vi "mp285_SetVelRes_velres2str.vi"(1 "速度":dbl, 2 "精度":u16(ring)=10 items=["Low (10microsteps/step)", "High (50microsteps/step)"]) -> (0 "发送至串口的字符串":string)   [LabVIEW 2018]
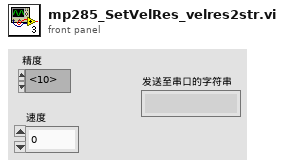
[diagram p1: front panel]
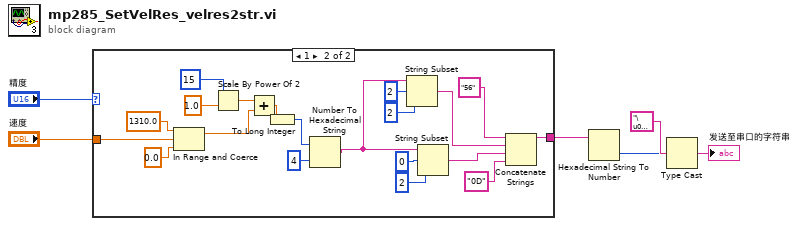
[diagram p0: block diagram]
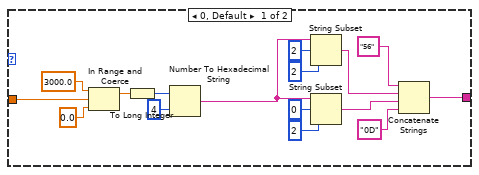
[diagram p2: hidden frame]
diagram:
  n1 = case shown="1" "精度" {
    tunnel: "速度" -> [w20 w42]
    tunnel: [w15 w30] -> w3
    frame 0, Default {
      n2 = In Range and Coerce(upper limit=3000.0 ("上限"), x=w20, lower limit=0.0 ("下限")) -> (coerced(x)=w19:dbl)  [unwired: 1 out]
      n3 = To Long Integer(number=w19) -> (32bit integer=w7:i32)
      n4 = Number To Hexadecimal String(1:i16 4 ("宽度(-)"), 2:w7) -> (0:w8:string)
      n5 = String Subset(string=w8, offset (0)=2 ("偏移量(0)"), length (rest)=2 ("长度（剩余）")) -> (substring=w10:string)
      n6 = String Subset(string=w8, offset (0)=0 ("偏移量(0)"), length (rest)=2 ("长度（剩余）")) -> (substring=w9:string)
      n7 = Concatenate Strings("56" ("字符串"), w10, w9, "0D" ("字符串")) -> (w15:string)
    }
    frame 1 {
      n8 = In Range and Coerce(upper limit=1310.0 ("上限"), x=w42, lower limit=0.0 ("下限")) -> (coerced(x)=w26:dbl)  [unwired: 1 out]
      n9 = Scale By Power Of 2(n=i16 15, x=1.0) -> (x*2^n=w27:dbl)
      n10 = Add(x=w27, y=w26) -> (x+y=w25:dbl)
      n11 = To Long Integer(number=w25) -> (32bit integer=w23:i32)
      n12 = Number To Hexadecimal String(1:i16 4 ("宽度(-)"), 2:w23) -> (0:w24:string)
      n13 = String Subset(string=w24, offset (0)=2 ("偏移量(0)"), length (rest)=2 ("长度（剩余）")) -> (substring=w32:string)
      n14 = String Subset(string=w24, offset (0)=0 ("偏移量(0)"), length (rest)=2 ("长度（剩余）")) -> (substring=w31:string)
      n15 = Concatenate Strings("56" ("字符串"), w32, w31, "0D" ("字符串")) -> (w30:string)
    }
  }
  n16 = Hexadecimal String To Number(string=w3) -> (number=w2:u32)  [unwired: 2 in, 1 out]
  n17 = Type Cast(type="\u0000", x=w2) -> (*(type *) &x=→"发送至串口的字符串":string)
